vi "ToWaveformChart.vi"(8 "error in":errorcluster, 11 "Generic in":refnum<class "Generic.lvclass">) -> (0 "error out":errorcluster, 3 "WFChart out":refnum<class "WaveformChart.lvclass">)   [LabVIEW 2014, in "Raspberry Pi Compatible Compiler for LabVIEW.lvlib" / "WaveformChart.lvclass"]
uses:
  WaveformChart.lvclass
  Generic/Generic.lvclass
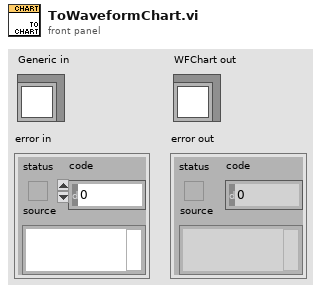
[diagram p1: front panel]
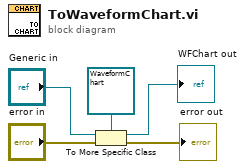
[diagram p0: block diagram]
diagram:
  n1 = To More Specific Class(target class=refnum<class "WaveformChart.lvclass"> refnum ("RotaryColorScale in 2"), reference="Generic in", error in="error in") -> (specific class reference=→"WFChart out":refnum<class "WaveformChart.lvclass">, error out=→"error out":errorcluster)
